vi "Voltage Read Array.vi"(11 "Device in":refnum<class "Device.lvclass">) -> (2 "Voltage.SP":dbl[](array[numeric]), 3 "Device out":refnum<class "Device.lvclass">)   [LabVIEW 2023, in "Device.lvclass"]
uses:
  Device.lvclass
  Device.lvclass/Device.ctl
  Low Level Capabilities/Voltage/Voltage Setpoint/Voltage Setpoint.lvclass
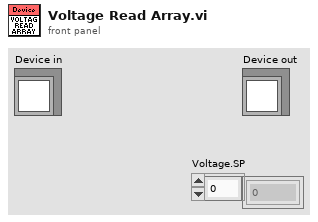
[diagram p1: front panel]
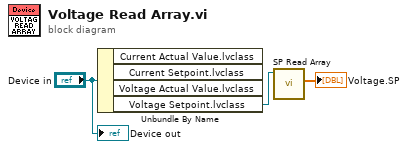
[diagram p0: block diagram]
diagram:
  n1 = Unbundle By Name("Device in") -> ("Voltage Setpoint.lvclass"=w1:refnum<class "Voltage Setpoint.lvclass">)  [unwired: 3 out]
  n2 = call-dynamic "SP Read Array.vi"("Voltage Setpoint.lvclass"=w1) -> ("Current Setpoint"=→"Voltage.SP":dbl[])  [unwired: 7 in, 3 out]
  "Device out" <- "Device in"
